vi "SUBVI_MDT693B_write_only-xyI.vi"(8 "error in (no error)":errorcluster, 9 "y":dbl, 10 "x":dbl, 11 "VISA Refnum in":refnum<visa-resource-name>) -> (0 "error out":errorcluster, 3 "VISA Refnum out":refnum<visa-resource-name>)   [LabVIEW 2020]
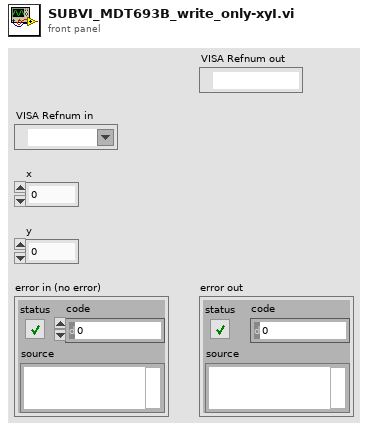
[diagram p1: front panel]
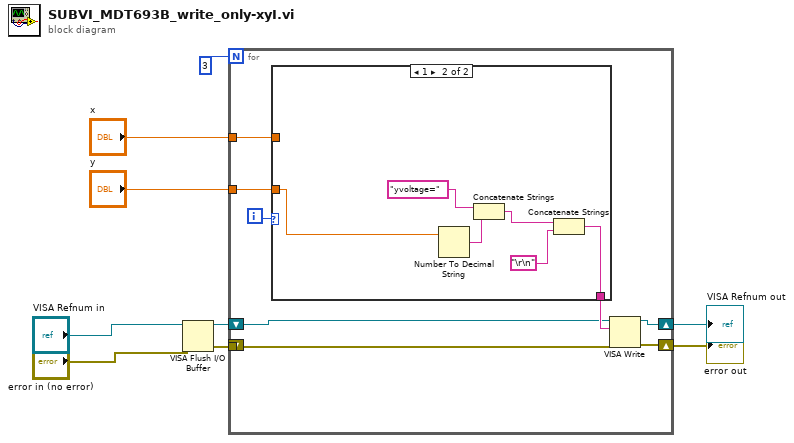
[diagram p0: block diagram]
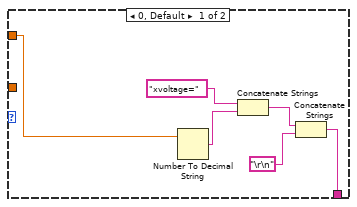
[diagram p2: hidden frame]
diagram:
  n1 = VISA Flush I/O Buffer(VISA resource name="VISA Refnum in", error in (no error)="error in (no error)") -> (VISA resource name out=w7:refnum<visa-resource-name>, error out=w6:errorcluster)  [unwired: 1 in]
  n2 = for {
    N: 3 -> [_]
    tunnel: w6 -> [w14]
    shift-right: [w13] -> w2
    shift-left: _ -> [_]
    shift-right: [w12] -> w3
    shift-left: w7 -> [w15]
    tunnel: "x" -> [w11]
    tunnel: "y" -> [w10]
    i -> [w17]
    n3 = case shown="1" w17 {
      tunnel: [w19 w25] -> w16
      tunnel: w11 -> [w18 _]
      tunnel: w10 -> [_ w24]
      frame 0, Default {
        n4 = Number To Decimal String(number=w18) -> (decimal integer string=w22:string)  [unwired: 1 in]
        n5 = Concatenate Strings("xvoltage=", w22) -> (w21:string)
        n6 = Concatenate Strings(w21, "\r\n") -> (w19:string)
      }
      frame 1 {
        n7 = Number To Decimal String(number=w24) -> (decimal integer string=w28:string)  [unwired: 1 in]
        n8 = Concatenate Strings("yvoltage=", w28) -> (w27:string)
        n9 = Concatenate Strings(w27, "\r\n") -> (w25:string)
      }
    }
    n10 = VISA Write(VISA resource name=w15, write buffer=w16, error in (no error)=w14) -> (VISA resource name out=w12:refnum<visa-resource-name>, error out=w13:errorcluster)  [unwired: 1 out]
  }
  "VISA Refnum out" <- w3
  "error out" <- w2
